vi "ABB CheckHasp_WPX_Std.vi"() -> (3 "Verified":bool)   [LabVIEW 2017]
panel:
  in  "Pass2":i32=21499
  in  "Pass1":i32=1985
  in  "Dialogs On":bool
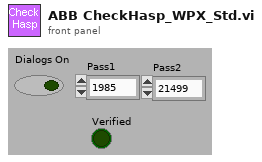
[diagram p1: front panel]
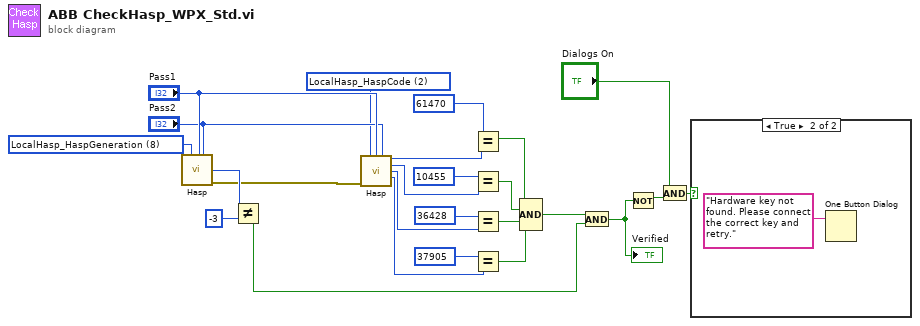
[diagram p0: block diagram]
diagram:
  w19 = u16 2 items=["LocalHasp_IsHasp"=1, "LocalHasp_HaspCode"=2, "LocalHasp_HaspStatus/API_Version"=5, "LocalHasp_HaspGeneration"=8, "LocalHasp_HaspNetStatus"=9, "LocalHasp_EncodeData"=60, "LocalHasp_DecodeData"=61, "NEtHasp_EncodeData"=88, "NetHasp_DecodeData"=89] ("Service")
  w25 = u16 8 items=["LocalHasp_IsHasp"=1, "LocalHasp_HaspCode"=2, "LocalHasp_HaspStatus/API_Version"=5, "LocalHasp_HaspGeneration"=8, "LocalHasp_HaspNetStatus"=9, "LocalHasp_EncodeData"=60, "LocalHasp_DecodeData"=61, "NEtHasp_EncodeData"=88, "NetHasp_DecodeData"=89] ("Service")
  n1 = call "Hasp.vi"("Service"=w25, "pass1"="Pass1", "pass2"="Pass2") -> ("param3"=w24:i32, "error out"=w22:errorcluster)  [unwired: 8 in, 3 out]
  n2 = Not Equal?(x=w24, y=-3) -> (x != y?=w5:bool)
  n3 = call "Hasp.vi"("Service"=w19, "pass1"="Pass1", "pass2"="Pass2", "error in (no error)"=w22) -> ("param1"=w18:i32, "param2"=w17:i32, "param3"=w16:i32, "param4"=w15:i32)  [unwired: 7 in, 1 out]
  n4 = Equal?(x=61470 ("param1"), y=w18) -> (x = y?=w12:bool)
  n5 = Equal?(x=10455, y=w17) -> (x = y?=w11:bool)
  n6 = Equal?(x=36428 ("param3"), y=w16) -> (x = y?=w10:bool)
  n7 = Equal?(x=37905 ("Param4"), y=w15) -> (x = y?=w9:bool)
  n8 = Compound Arithmetic op=AND(w12, w11, w10, w9) -> (w6:bool)
  n9 = And(x=w6, y=w5) -> (x .and. y?=w4:bool)
  "Verified" <- w4
  n10 = Not(x=w4) -> (.not. x?=w3:bool)
  n11 = And(x="Dialogs On", y=w3) -> (x .and. y?=w1:bool)
  n12 = case shown="True" w1 {
    frame False {
    }
    frame True {
      n13 = One Button Dialog(message="Hardware key not found. Please connect the correct key and retry.") -> ()  [unwired: 1 in, 1 out]
    }
  }
